vi "RAM_MB Available.vi"(8 "Error":errorcluster, 9 "Close":bool, 11 "New Ref":refnum<k24>) -> (0 "Error Out":errorcluster, 2 "MB Of Avalible Ram Out":sgl, 3 "New Ref Out":refnum<k24>)   [LabVIEW 2015]
doc: "Get the availible Ram using .net"
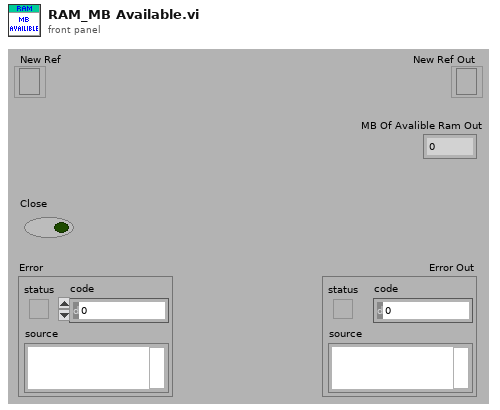
[diagram p1: front panel]
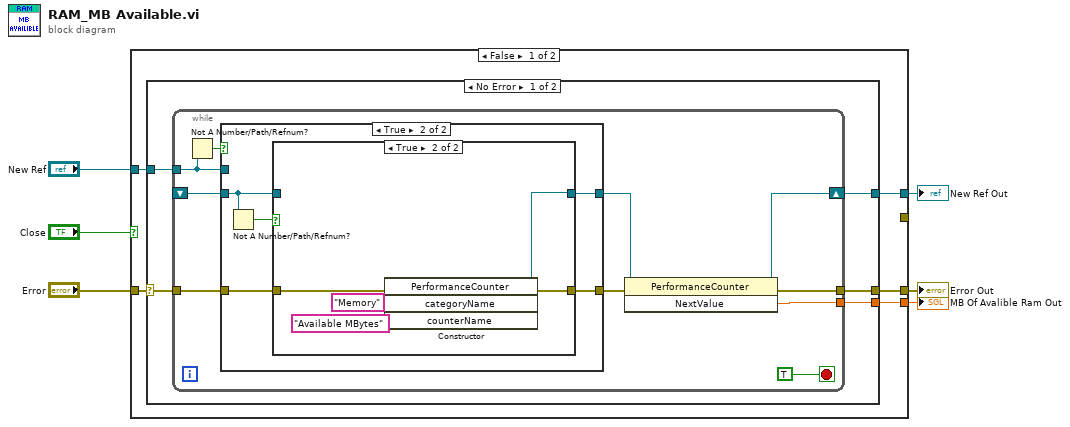
[diagram p0: block diagram]
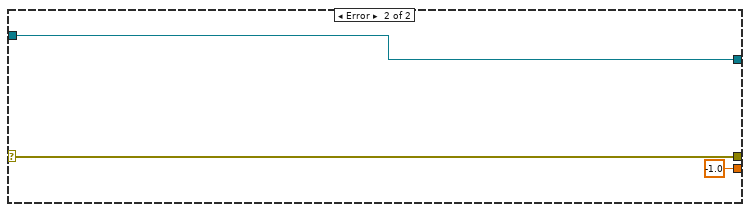
[diagram p4: hidden frame]
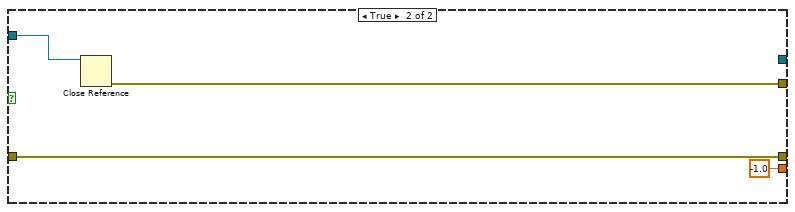
[diagram p5: hidden frame]
diagram:
  n1 = case shown="False" "Close" {
    tunnel: [w11 w45] -> w6
    tunnel: [w10 sgl -1.0 ("NextValue")] -> w5
    tunnel: "New Ref" -> [w9 w47]
    tunnel: [w8 _] -> w1
    tunnel: "Error" -> [w7 w45]
    tunnel: [_ w46] -> _
    frame False {
      n2 = case shown="No Error" w7 {
        selector: w7 -> [w13 w42]
        tunnel: [w16 w42] -> w11
        tunnel: [w15 sgl -1.0 ("NextValue")] -> w10
        tunnel: w9 -> [w12 w43]
        tunnel: [w14 w43] -> w8
        frame No Error {
          n3 = while {
            tunnel: [w24] -> w16
            tunnel: [w23] -> w15
            tunnel: w13 -> [w19]
            shift-right: [w20] -> w14
            shift-left: _ -> [w21]
            tunnel: w12 -> [w18]
            stop <- TRUE stop-if-true
            n4 = Not A Number/Path/Refnum?(number/path/refnum=w18) -> (NaN/Path/Refnum?=w22:bool)
            n5 = case shown="True" w22 {
              tunnel: [w27 w33] -> w26
              tunnel: [w28 w32] -> w25
              tunnel: w19 -> [w28 w31]
              tunnel: w21 -> [_ w29]
              tunnel: w18 -> [w27 _]
              frame False {
              }
              frame True {
                n6 = Not A Number/Path/Refnum?(number/path/refnum=w29) -> (NaN/Path/Refnum?=w30:bool)
                n7 = case shown="True" w30 {
                  tunnel: [w35 w36] -> w33
                  tunnel: [w34 w38] -> w32
                  tunnel: w31 -> [w34 w37]
                  tunnel: w29 -> [w35 _]
                  frame False {
                  }
                  frame True {
                    n8 = constructor class="PerformanceCounter"(error in=w37, "categoryName"="Memory", "counterName"="Available MBytes") -> (reference out=w36:refnum<k24>, error out=w38:errorcluster)  [unwired: 2 in, 3 out]
                  }
                }
              }
            }
            n9 = invoke class="PerformanceCounter" method="NextValue"(reference=w26, error in=w25) -> (reference out=w20:refnum<k24>, error out=w24:errorcluster, "NextValue"=w23:sgl)  [unwired: 1 in]
          }
        }
        frame Error {
        }
      }
    }
    frame True {
      n10 = Close Reference(reference=w47) -> (error out=w46:errorcluster)  [unwired: 1 in]
    }
  }
  "Error Out" <- w6
  "MB Of Avalible Ram Out" <- w5
  "New Ref Out" <- w1
